vi "Control Mode Write Single.vi"(8 "error in":errorcluster, 9 "Channel Index":i32, 10 "Control Mode STS":u16, 11 "Cycler in":refnum<class "Cycler.lvclass">) -> (0 "error out":errorcluster, 3 "Cycler out":refnum<class "Cycler.lvclass">)   [LabVIEW 2023, in "Cycler.lvclass"]
uses:
  Cycler.lvclass
  Cycler.lvclass/Cycler.ctl
  Low Level Capabilities/Control Mode/Control Mode.lvclass
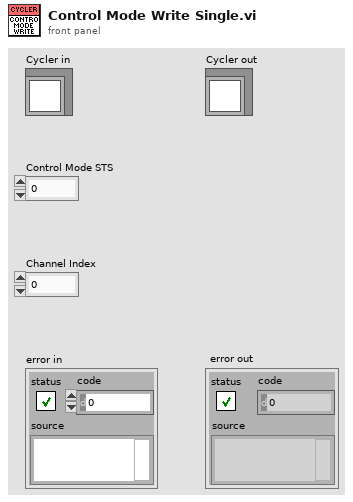
[diagram p1: front panel]
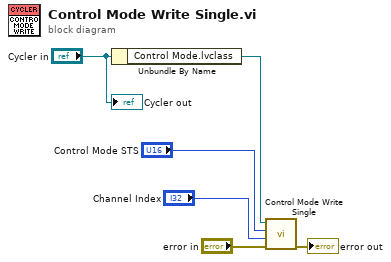
[diagram p0: block diagram]
diagram:
  n1 = Unbundle By Name("Cycler in") -> ("Control Mode.lvclass"=w6:refnum<class "Control Mode.lvclass">)
  n2 = call-dynamic "Control Mode Write Single.vi"("error in"="error in", "Channel Index"="Channel Index", "Control Mode STS"="Control Mode STS", "Control Mode in"=w6) -> ("error out"=→"error out":errorcluster)  [unwired: 6 in, 1 out]
  "Cycler out" <- "Cycler in"
